vi "Stim Train_new.vi"(4 "Single Channel Params":T1 {"Train Length" min=20 max=500 step=5}, 5 "Stimulator":T2={"Stim Open Data"={"Name"="", "Mode"=enum."LIVE", "Visa Timeout"=0}, "Stim Init Data"={"Frequency"=0.0, "N Factor"=0, "D/T Int"=0.0, "Active Channels"=[], "LF Channels"=[]}, "Stim Update Data"={"Pulse Mode"=[enum."Single"], "Current"=[], "Pulse Dur"=[]}, "Stim Status"={"Open"=FALSE, "On"=FALSE}}) -> (1 "Stim Train Log String":string, 2 "Stimulator Out":T2={"Stim Open Data"={"Name"="", "Mode"=enum."LIVE", "Visa Timeout"=0}, "Stim Init Data"={"Frequency"=0.0, "N Factor"=0, "D/T Int"=0.0, "Active Channels"=[], "LF Channels"=[]}, "Stim Update Data"={"Pulse Mode"=[enum."Single"], "Current"=[], "Pulse Dur"=[]}, "Stim Status"={"Open"=FALSE, "On"=FALSE}})   [LabVIEW 2019]
uses:
  Data Type Defs/Stimulator.ctl
  Data Type Defs/Stim Open Data.ctl
  Data Type Defs/Stim Init Data.ctl
  Data Type Defs/Stim Update Data.ctl
  Data Type Defs/Pulse Mode (array).ctl
  Data Type Defs/Stim Status.ctl
  Controls/Type Defs/Single Channel Params.ctl
panel:
  out "Log Entry":string
  out "Write to Log 2":string
  out "Write to Log":string
  out "Actual Train Length":u32
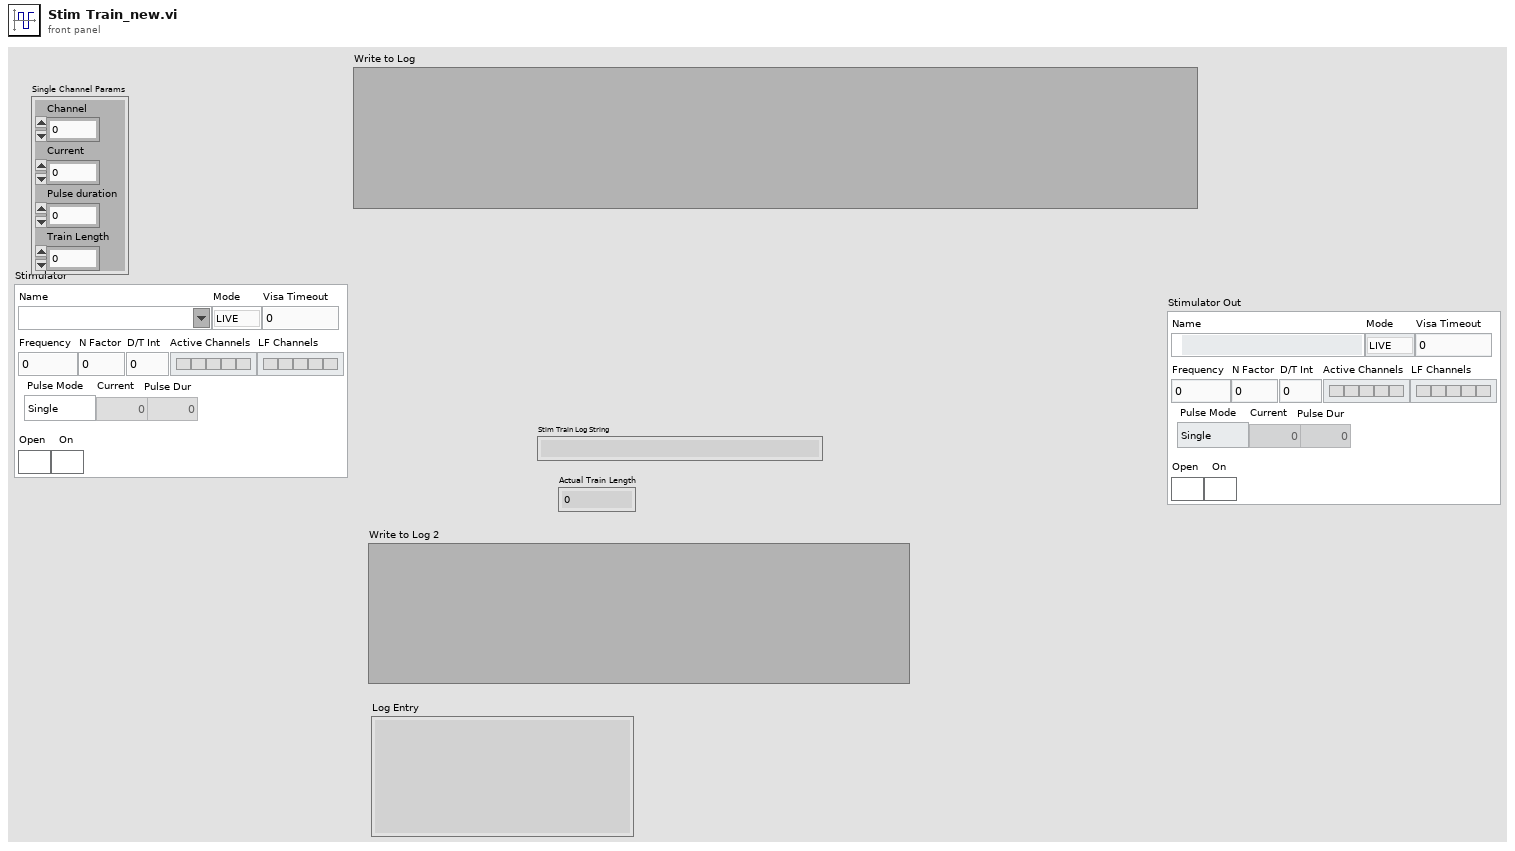
[diagram p1: front panel]
types:
  T1 = typedef "Single Channel Params.ctl" = cluster{"Channel":i32, "Current":u8, "Pulse duration":u16, "Train Length":i64}
  T2 = typedef "Stimulator.ctl" = cluster{"Stim Open Data":T3, "Stim Init Data":T4, "Stim Update Data":T5, "Stim Status":T7}
  T3 = typedef "Stim Open Data.ctl" = cluster{"Name":refnum<visa-resource-name>, "Mode":enum16{"LIVE", "SIM"}, "Visa Timeout":u32}
  T4 = typedef "Stim Init Data.ctl" = cluster{"Frequency":dbl, "N Factor":u8, "D/T Int":dbl, "Active Channels":bool[], "LF Channels":bool[]}
  T5 = typedef "Stim Update Data.ctl" = cluster{"Pulse Mode":T6, "Current":u32[], "Pulse Dur":u32[]}
  T6 = typedef "Pulse Mode (array).ctl" = enum16{"Single", "Doublet", "Triplet"}[]
  T7 = typedef "Stim Status.ctl" = cluster{"Open":bool, "On":bool}
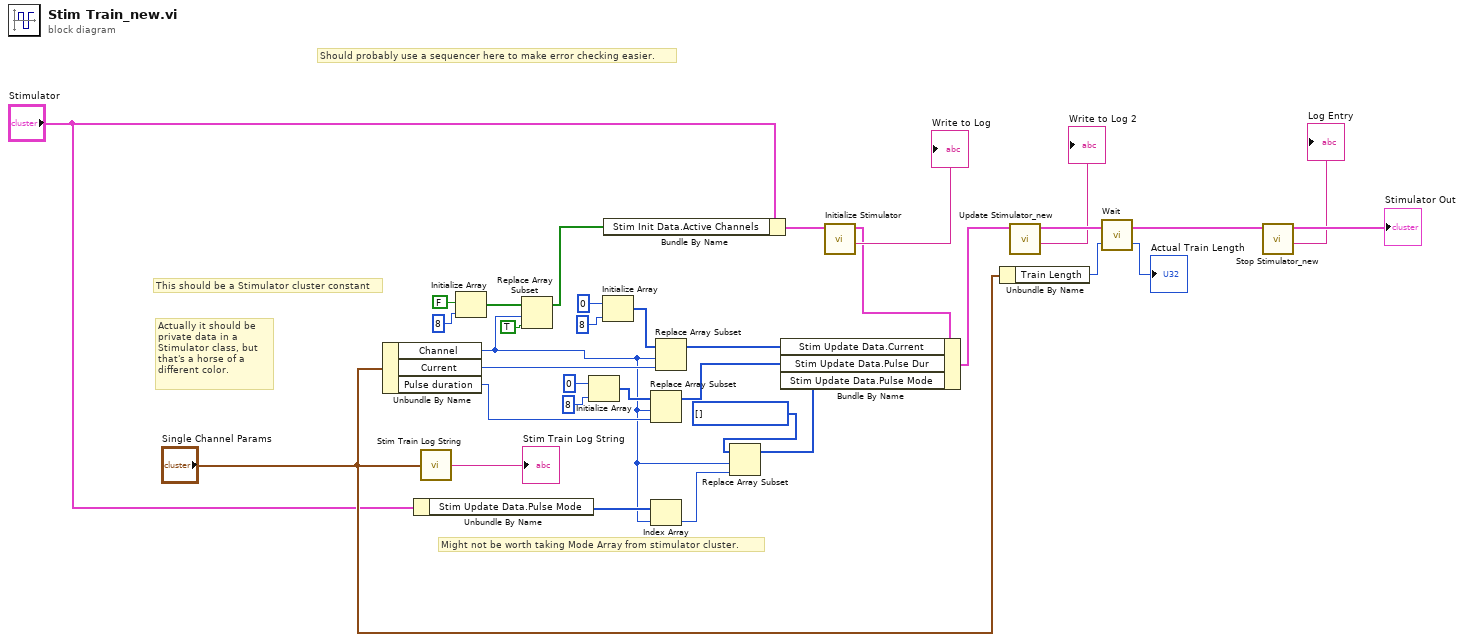
[diagram p0: block diagram]
diagram:
  w6 = enum16{"Single", "Doublet", "Triplet"}[] [] items=["Single", "Doublet", "Triplet"] ("output array")
  # "Might not be worth taking Mode Array from stimulator cluster."
  # "Actually it should be private data in a Stimulator class, but that's a horse of a different color."
  # "This should be a Stimulator cluster constant"
  # "Should probably use a sequencer here to make error checking easier."
  n1 = Unbundle By Name("Single Channel Params") -> ("Channel"=w14:i32, "Current"=w28:u8, "Pulse duration"=w16:u16)
  n2 = Unbundle By Name("Stimulator") -> ("Stim Update Data.Pulse Mode"=w15:T6)
  n3 = call "Stim Train Log String.vi"("Single Channel Params"="Single Channel Params") -> ("Stim Train Log String"=→"Stim Train Log String":string)
  n4 = Initialize Array(FALSE, 8 ("dimension size")) -> (w30:bool[])
  n5 = Replace Array Subset(array=w30, new element=TRUE ("new element/subarray"), index=w14) -> (w1:bool[])
  n6 = Initialize Array(u8 0 ("dimension size"), 8 ("dimension size")) -> (w23:u8[])
  n7 = Initialize Array(u8 0 ("dimension size"), 8 ("dimension size")) -> (w27:u8[])
  n8 = Bundle By Name(cluster="Stimulator", "Stim Init Data.Active Channels"=w1) -> (w2:T2)
  n9 = Replace Array Subset(array=w23, new element=w16, index=w14) -> (w17:u8[])
  n10 = Index Array(array=w15, index=w14) -> (element=w13:enum16{"Single", "Doublet", "Triplet"})
  n11 = Replace Array Subset(array=w27, new element=w28, index=w14) -> (w18:u8[])
  n12 = Replace Array Subset(array=w6, new element=w13, index=w14) -> (w5:enum16{"Single", "Doublet", "Triplet"}[])
  n13 = call "Initialize Stimulator.vi"("Stimulator"=w2) -> ("Write to Log"=→"Write to Log":string, "Stimulator"=w7:T2)  [unwired: 3 in, 2 out]
  n14 = Bundle By Name(cluster=w7, "Stim Update Data.Current"=w18, "Stim Update Data.Pulse Dur"=w17, "Stim Update Data.Pulse Mode"=w5) -> (w4:T2)
  n15 = Unbundle By Name("Single Channel Params") -> ("Train Length"=w11:i64)
  n16 = call "Update Stimulator_new.vi"("Stimulator"=w4) -> ("Write to Log"=→"Write to Log 2":string, "Stimulator"=w20:T2)  [unwired: 3 in, 2 out]
  n17 = call "Wait.vi"("milliseconds to wait"=w11, "Stimulator"=w20) -> ("Milliseconds Waited"=→"Actual Train Length":u32, "Stimulator"=w19:T2)
  n18 = call "Stop Stimulator_new.vi"("Stimulator"=w19) -> ("Log Entry"=→"Log Entry":string, "Stimulator Out"=→"Stimulator Out":T2)  [unwired: 3 in, 2 out]
